vi "ADXL335Simulator2025.vi"(3 "Loop count":i32, 4 "CPR?":bool, 5 "loop period, msec in":u32=200) -> ()   [LabVIEW 2023]
panel:
  out "output variable":dbl[](array[numeric])
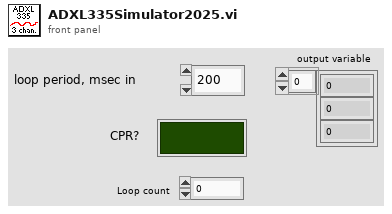
[diagram p1: front panel]
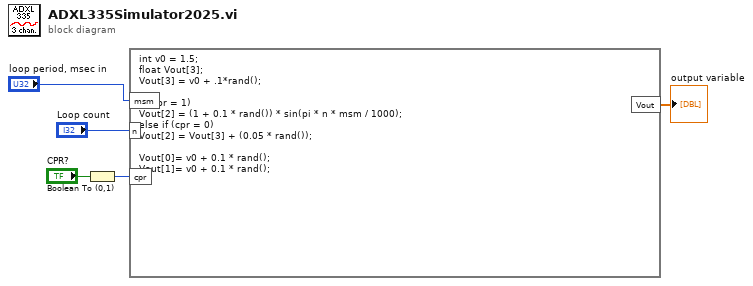
[diagram p0: block diagram]
diagram:
  n1 = Boolean To (0,1)(Boolean="CPR?") -> (0, 1=w3:i16)
  n2 = formula code="int v0 = 1.5;\nfloat Vout[3];\nVout[3] = v0 + .1*rand();\n\nif (cpr = 1)\nVout[2] = (1 + 0.1 * rand()) * sin(pi * n * msm / 1000);\nelse if (cpr = 0)\nVout[2] = Vout[3] + (0.05 * rand());\n\nVout[0]= v0 + 0.1 * rand();  \nVout[1]= v0 + 0.1 * rand();"("msm"="loop period, msec in", "n"="Loop count", "cpr"=w3) -> ("Vout"=→"output variable":dbl[])
